vi "ui_DataLog Query New Value.vi"(7 "tag info":T1 {"logging parameters" format="%.2e"; "precision" items=["0", "1", "2", "3", "4", "5", "6", "7", "8", "9", "10", "11", "12", "13", "14", "15", "16", "17"]; "limit delay" format="%.2e"; "deadband" format="%.2e"}) -> (4 "OKed?":bool, 8 "new value out":dbl format="%.2f")   [LabVIEW 2012]
doc: "This dialog queries for a new tag value and sets it when OKed."
uses:
  typedefs/clusters/t_DataLog Tag Config.ctl
  typedefs/t_DataLog Temporal Types.ctl
  typedefs/t_DataLog Value Types.ctl
  typedefs/t_DataLog Numerical Format.ctl
  typedefs/t_DataLog Logging Algorithms.ctl
  typedefs/t_DataLog Query New Value States.ctl
panel:
  in  "new value":dbl format="%.4e"
  in  "cancel":bool
  in  "OK":bool
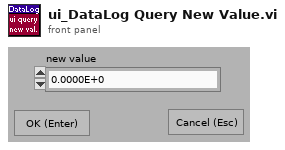
[diagram p1: front panel]
types:
  T1 = typedef "t_DataLog Tag Config.ctl" = cluster{"name":string, "unit":string, "temporal":T2, "value":T3, "index":i32, "capacity":i32, "is meta?":bool, "mincapacity":i32, "deadband":dbl, "limit delay":dbl, "format":T4, "precision":u8, "undefine":bool, "update":bool, "update period":u16, "expression":string, "description":string, "logging algorithm":T5, "logging parameters":dbl[]}
  T2 = typedef "t_DataLog Temporal Types.ctl" = enum16{"set&hold", "sample", "event"}
  T3 = typedef "t_DataLog Value Types.ctl" = enum16{"number", "string"}
  T4 = typedef "t_DataLog Numerical Format.ctl" = enum8{"fractional", "exponential", "engineering"}
  T5 = typedef "t_DataLog Logging Algorithms.ctl" = enum16{"nothing", "changes", "everything", "every Nth", "time threshold", "value threshold + prior", "t or v threshold", "t or v threshold + prior"}
  T6 = typedef "t_DataLog Query New Value States.ctl" = enum16{"empty queue", "initialize", "stop"}
  T7 = typedef "eventvkey.ctl" = enum16{"ASCII", "Enter", "Return", "Shift", "Ctrl", "Alt", "Cmd", "Opt", "Caps", "NumLock", "Clear", "Break", "Up", "Down", "Left", "Right", "Insert", "Delete", "Home", "End", "PageUp", "PageDown", "Escape", "Help", "Pause", "ScrollLock", "F1", "F2", "F3", "F4", "F5", "F6", "F7", "F8", "F9", "F10", "F11", "F12", "F13", "F14", "F15", "F16", "F17", "F18", "F19", "F20", "F21", "F22", "F23", "F24", "Play", "VolumeUp", "VolumeDown", "Mute", "Two Byte Char"}
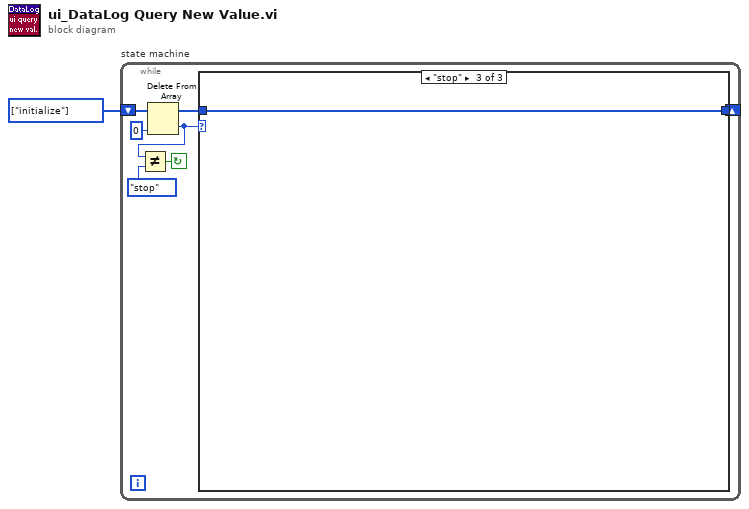
[diagram p0: block diagram]
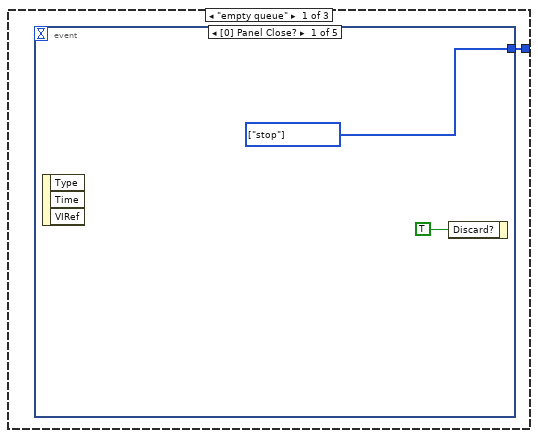
[diagram p2: hidden frame]
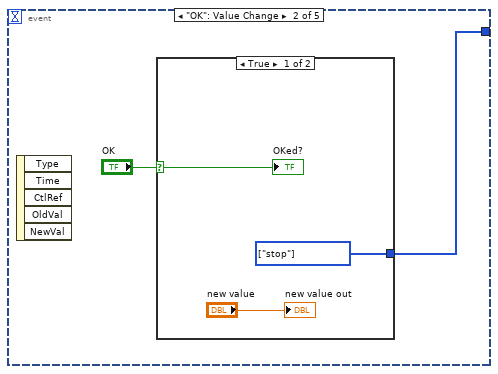
[diagram p3: hidden frame]
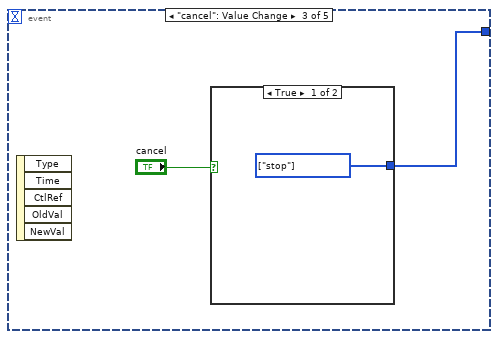
[diagram p5: hidden frame]
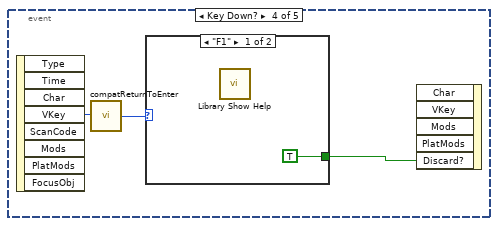
[diagram p7: hidden frame]
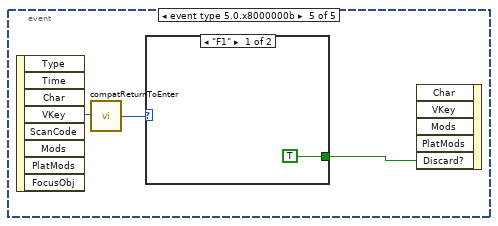
[diagram p9: hidden frame]
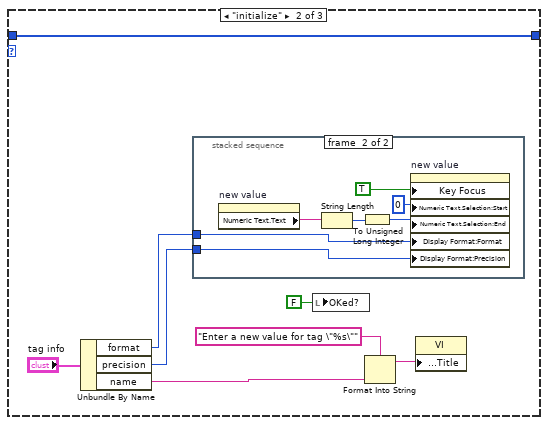
[diagram p11: hidden frame]
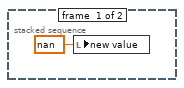
[diagram p12: hidden frame]
diagram:
  w1 = T6[] [enum."initialize"] items=["empty queue", "initialize", "stop"] ("Array Constant")
  n1 = while "state machine" {
    shift-left: w1 -> [w5]
    shift-right: [w8] -> _
    stop <- w7 continue-if-true
    n2 = Delete From Array(array=w5, index=0) -> (deleted portion=w3:T6, array with subset deleted=w4:T6[])  [unwired: 1 in]
    n3 = Not Equal?(x=w3, y=t_DataLog_Query_New_Value_States."stop" ("states")) -> (x != y?=w7:bool)
    n4 = case "Case" shown="\"stop\"" w3 {
      tunnel: [w9 w35 w44] -> w8
      tunnel: w4 -> [_ w35 w44]
      frame "empty queue" {
        n5 = event shown="[0] Panel Close?" {
          selector: _ -> [_ _ _ _ _]
          dyn-events: _ -> [_ _ _ _ _]
          timeout: _ -> [_ _ _ _ _]
          tunnel: [w11 w13 w18 _ _] -> w9
          event Panel Close? {
            w11 = T6[] [enum."stop"] items=["empty queue", "initialize", "stop"] ("Array Constant")
            n6 = event-data() -> ()  [unwired: 1 in, 3 out]
            n7 = event-data("Discard?"=TRUE) -> ()  [unwired: 1 in, 1 out]
          }
          event "OK": Value Change {
            n8 = event-data() -> ()  [unwired: 1 in, 5 out]
            n9 = case shown="True" "OK" {
              selector: "OK" -> [w15 _]
              tunnel: [w16 _] -> w13
              frame True {
                w16 = T6[] [enum."stop"] items=["empty queue", "initialize", "stop"] ("Array Constant")
                "OKed?" <- w15
                "new value out" <- "new value"
              }
              frame False {
              }
            }
          }
          event "cancel": Value Change {
            n10 = event-data() -> ()  [unwired: 1 in, 5 out]
            n11 = case shown="True" "cancel" {
              tunnel: [w19 _] -> w18
              frame True {
                w19 = T6[] [enum."stop"] items=["empty queue", "initialize", "stop"] ("Array Constant")
              }
              frame False {
              }
            }
          }
          event Key Down? {
            n12 = event-data() -> ("VKey"=w20:T7)  [unwired: 1 in, 7 out]
            n13 = call <vilib>:"compatReturnToEnter.vi"("VKey"=w20) -> ("VKey"=w22:T7)
            n14 = case shown="\"F1\"" w22 {
              tunnel: [TRUE ("Discard?") _] -> w21
              frame "F1" {
                n15 = call "Library Show Help.vi"() -> ()  [unwired: 1 in]
              }
              frame Default {
              }
            }
            n16 = event-data("Discard?"=w21) -> ()  [unwired: 5 in, 1 out]
          }
          event event type 5.0.x8000000b {
            n17 = event-data() -> ("VKey"=w24:T7)  [unwired: 1 in, 7 out]
            n18 = call <vilib>:"compatReturnToEnter.vi"("VKey"=w24) -> ("VKey"=w26:T7)
            n19 = case shown="\"F1\"" w26 {
              tunnel: [TRUE ("Discard?") _] -> w25
              frame "F1" {
              }
              frame Default {
              }
            }
            n20 = event-data("Discard?"=w25) -> ()  [unwired: 5 in, 1 out]
          }
        }
      }
      frame "initialize" {
        n21 = Unbundle By Name("tag info") -> ("format"=w29:T4, "precision"=w28:u8, "name"=w30:string)
        n22 = stacked-sequence {
          tunnel: w29 -> [_ w38]
          tunnel: w28 -> [_ w37]
          frame #0 {
            n23 = local write "new value"(nan ("initial value")) -> ()
          }
          frame #1 {
            n24 = property on="new value" class="DigNum (strict)"() -> ("Numeric Text.Text"=w41:string)  [unwired: 2 in, 2 out]
            n25 = String Length(string=w41) -> (length=w42:i32)
            n26 = To Unsigned Long Integer(number=w42) -> (unsigned 32bit integer=w40:u32)
            n27 = property on="new value" class="DigNum (strict)"("Key Focus"=TRUE, "Numeric Text.Selection:Start"=u32 0, "Numeric Text.Selection:End"=w40, "Display Format:Format"=w38, "Display Format:Precision"=w37) -> ()  [unwired: 2 in, 2 out]
          }
        }
        n28 = local write "OKed?"(FALSE ("OKed?")) -> ()
        n29 = Format Into String(format string="Enter a new value for tag \"%s\"", w30) -> (resulting string=w33:string)  [unwired: 2 in, 1 out]
        n30 = property class="VI"("Front Panel Window:Title"=w33) -> ()  [unwired: 2 in, 2 out]
      }
      frame "stop" {
      }
    }
  }
